vi "生成出厂配置.vi"(8 "error in":errorcluster) -> (0 "error out":errorcluster, 2 "ture?":bool)   [LabVIEW 2016]
panel:
  out "Numeric":i32
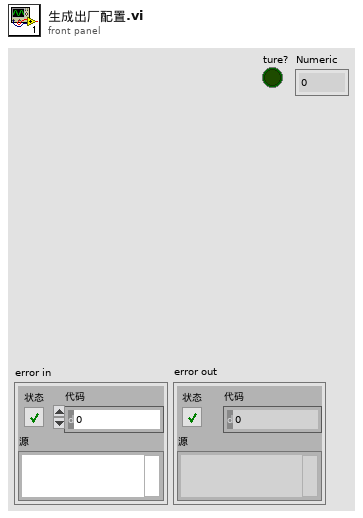
[diagram p1: front panel]
types:
  T1 = cluster{"byCmdType":u8, "bySubCmd":u8, "byPara":u8, "byAddr_h":u8, "byAddr_l":u8, "byAddr_ll":u8, "byLen_h":u8, "byLen_l":u8}
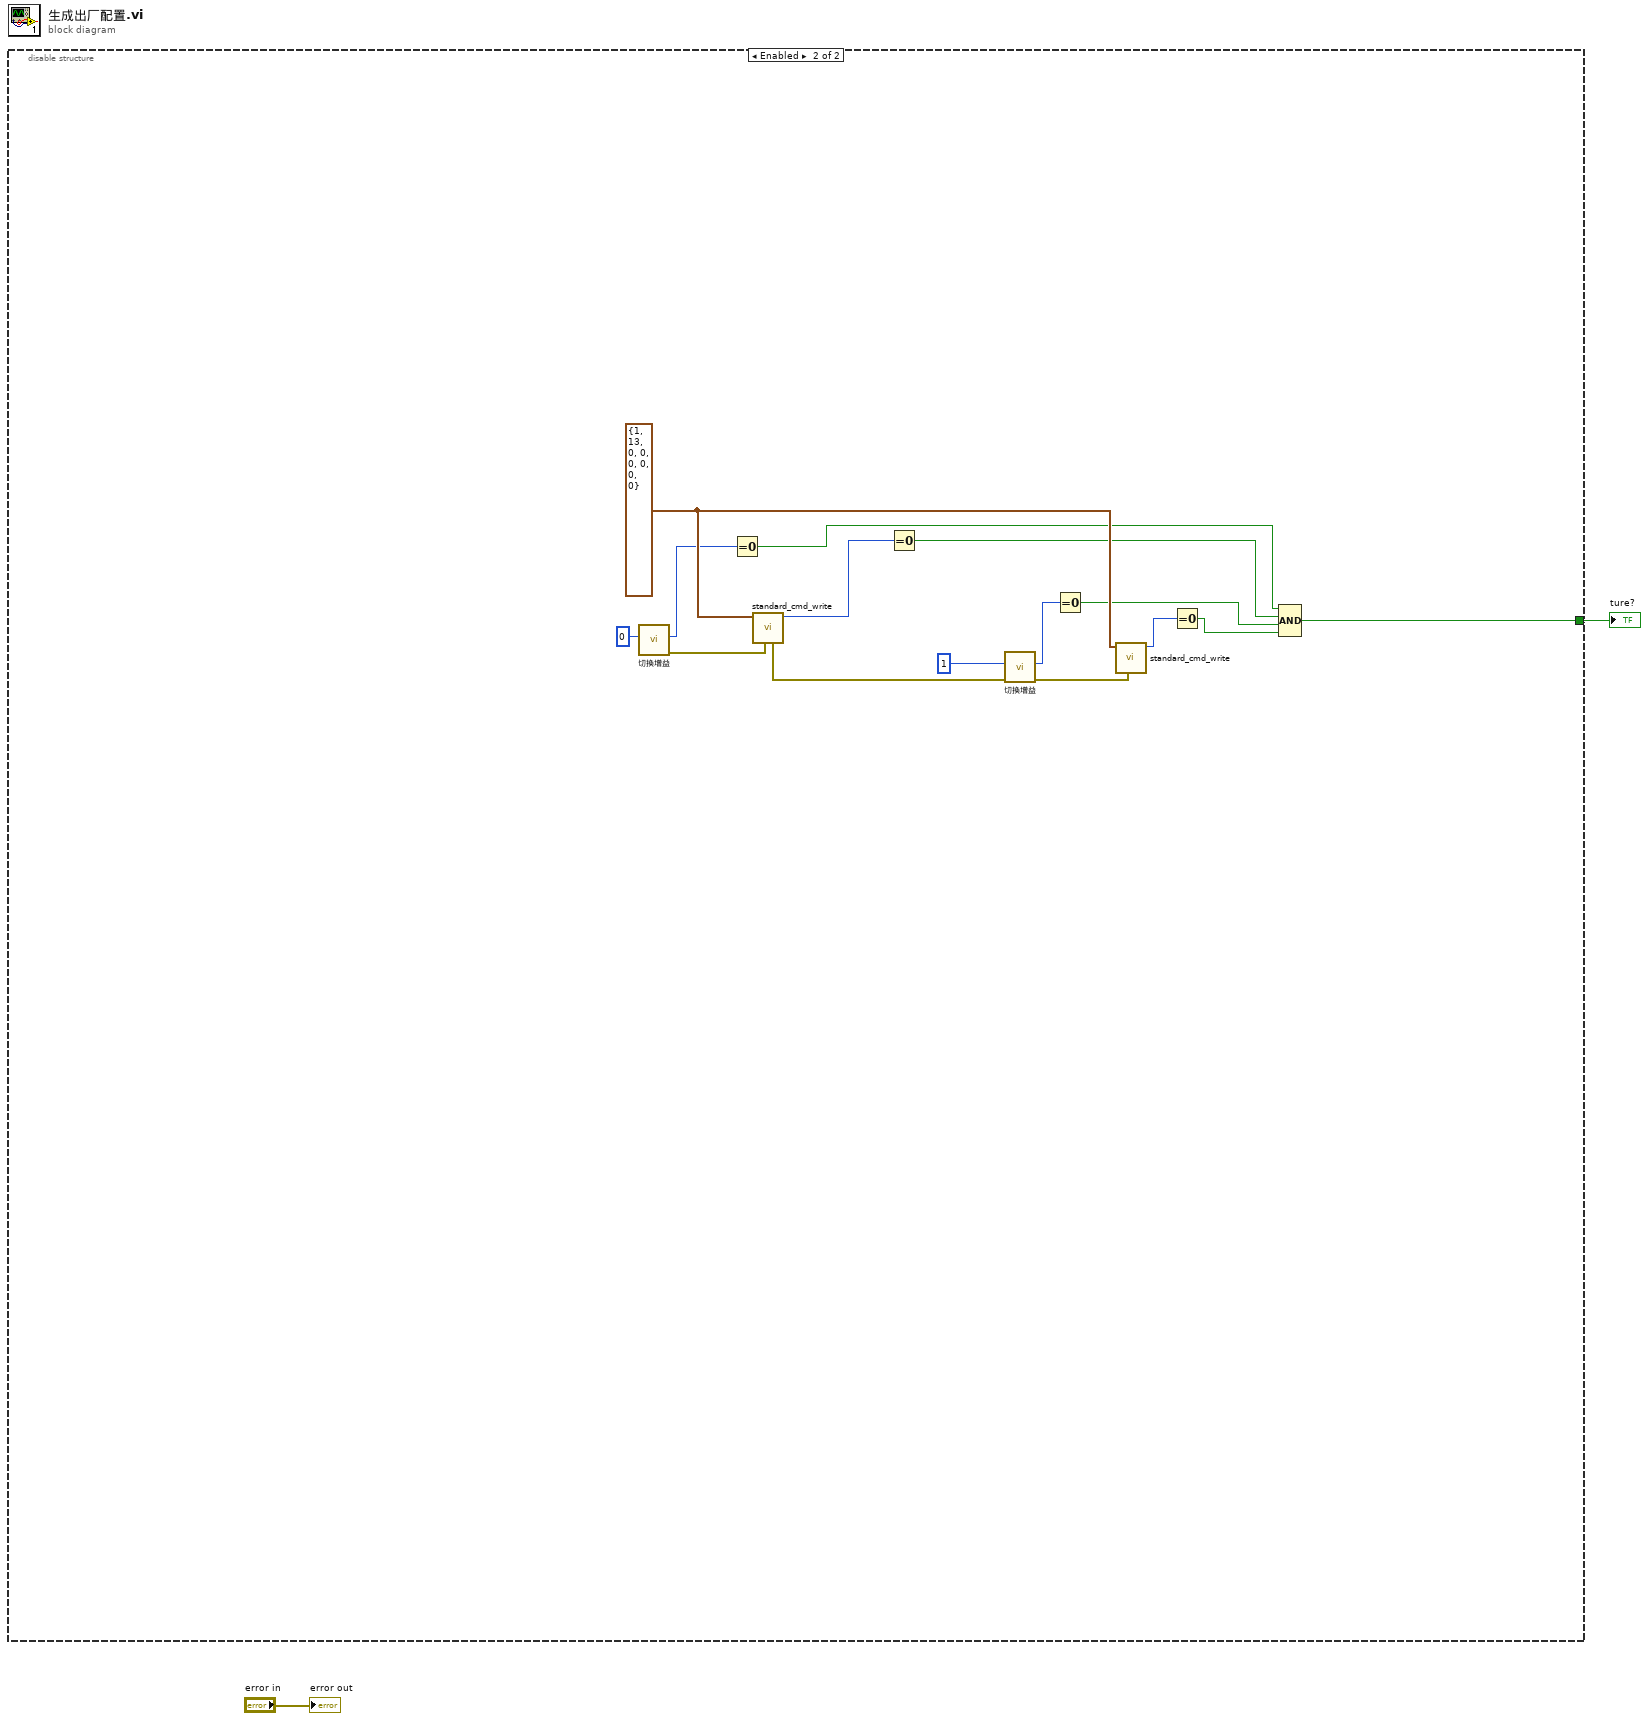
[diagram p0: block diagram]
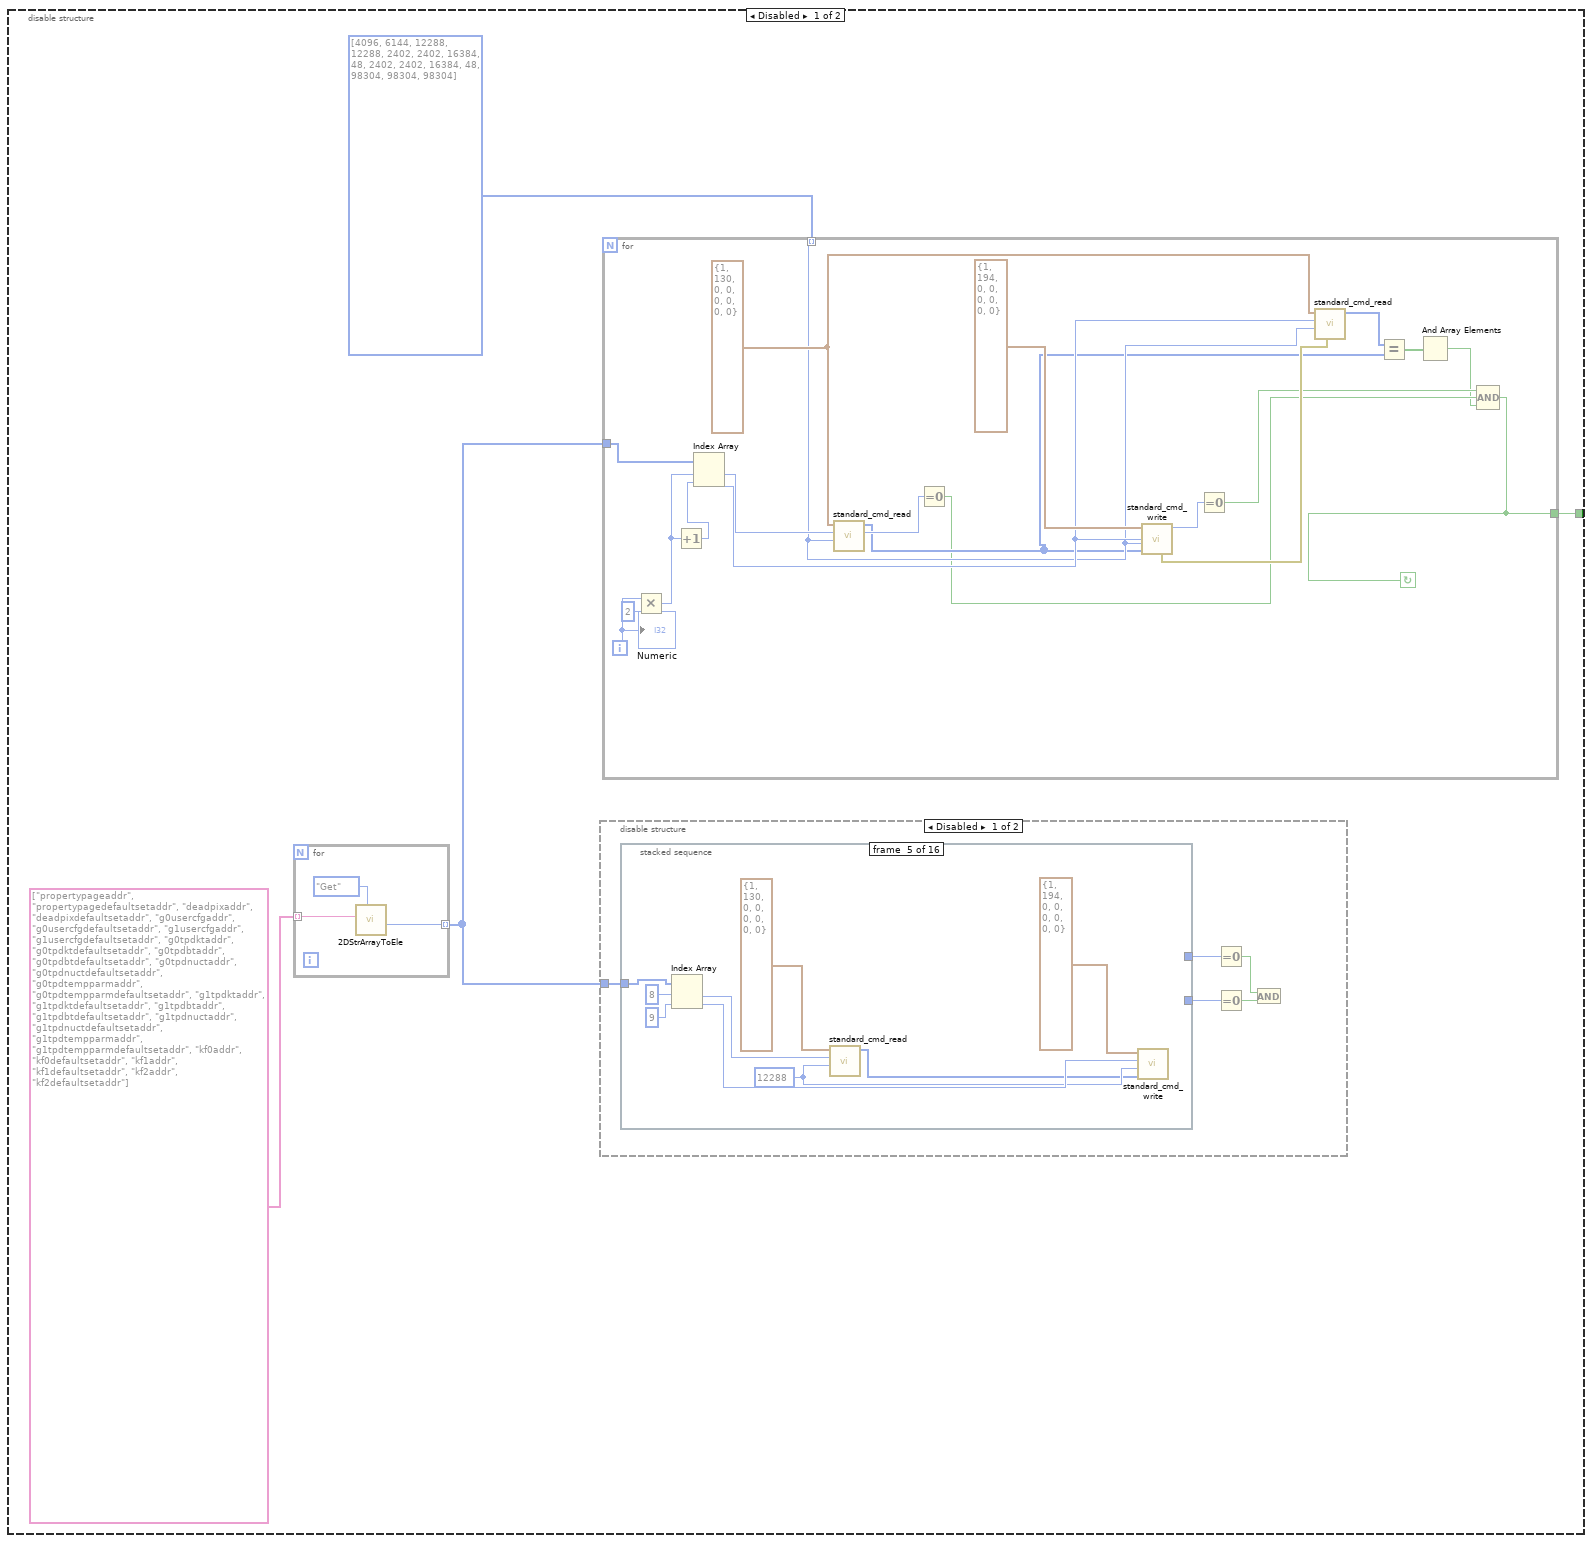
[diagram p2: hidden frame]
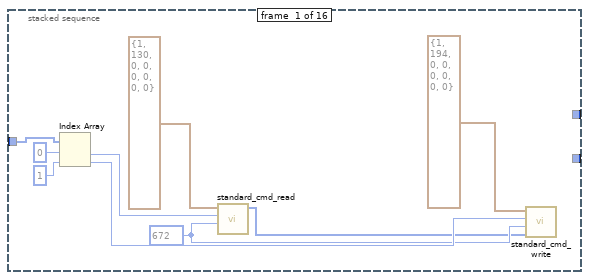
[diagram p3: hidden frame]
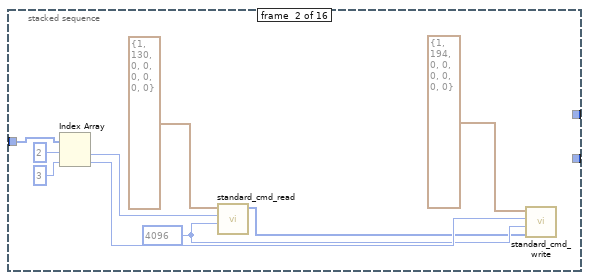
[diagram p4: hidden frame]
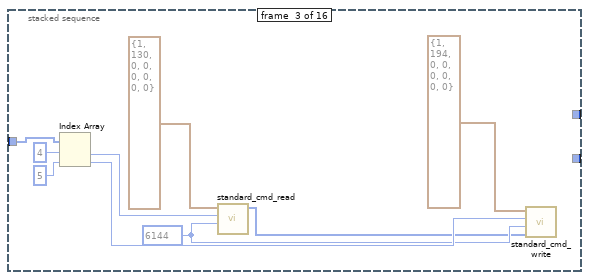
[diagram p5: hidden frame]
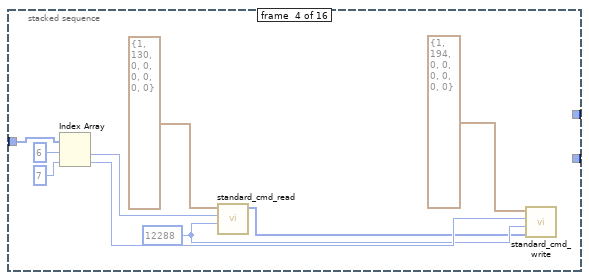
[diagram p6: hidden frame]
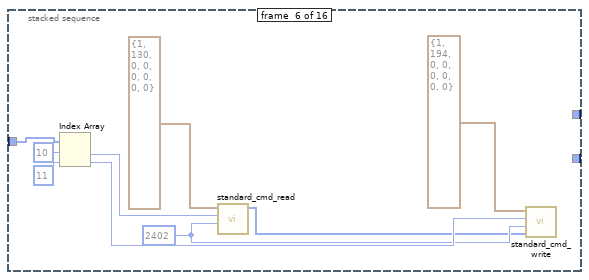
[diagram p7: hidden frame]
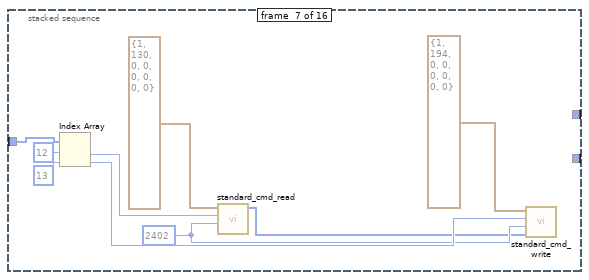
[diagram p8: hidden frame]
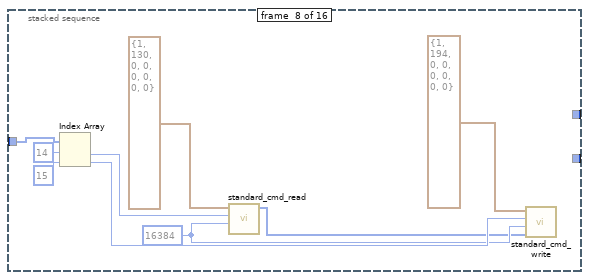
[diagram p9: hidden frame]
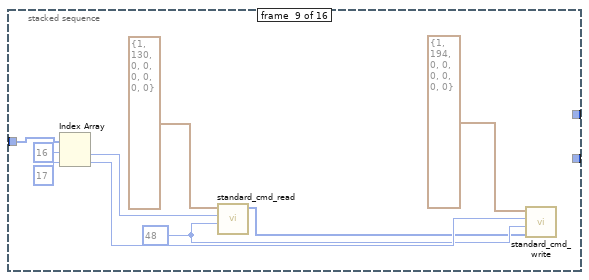
[diagram p10: hidden frame]
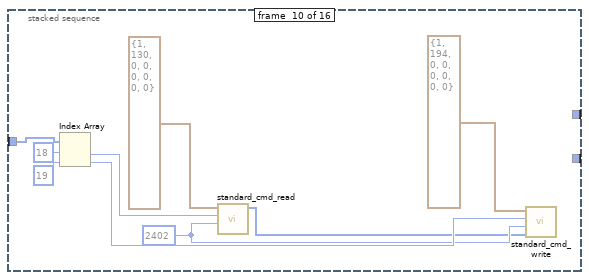
[diagram p11: hidden frame]
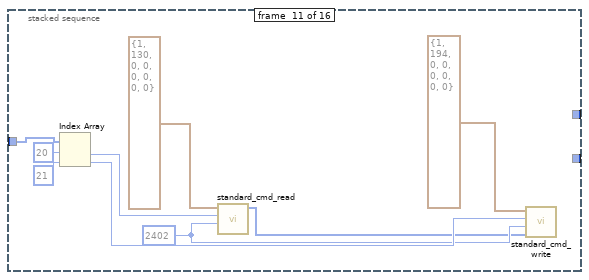
[diagram p12: hidden frame]
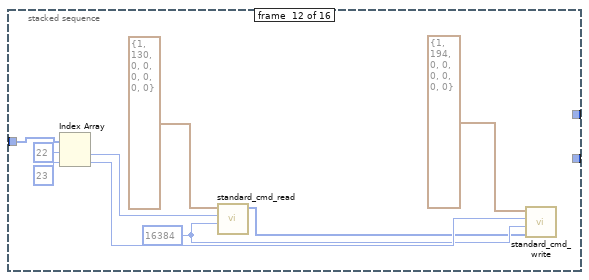
[diagram p13: hidden frame]
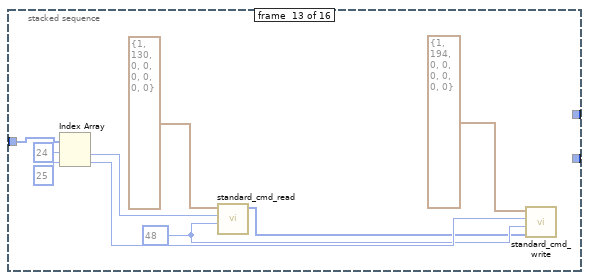
[diagram p14: hidden frame]
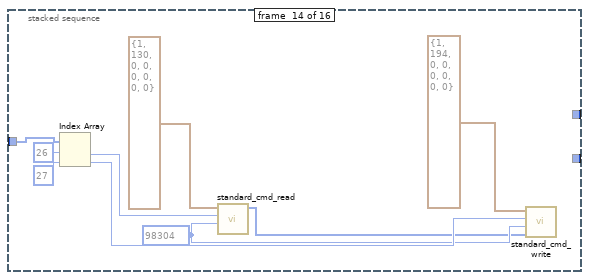
[diagram p15: hidden frame]
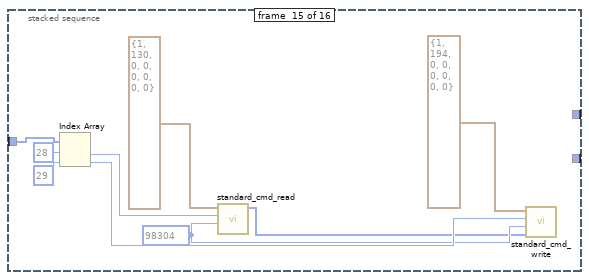
[diagram p16: hidden frame]
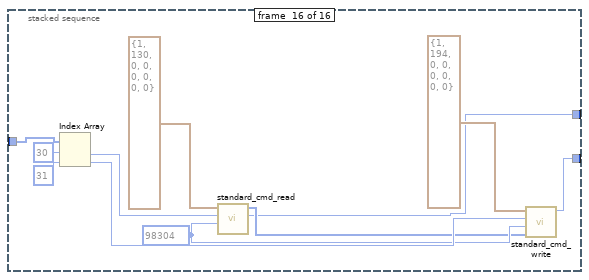
[diagram p17: hidden frame]
diagram:
  n1 = disable-structure shown="Enabled" {
    disable-tunnel: [w3 w181] -> w2
    frame Disabled {
      n2 = for {
        tunnel: string[] ["propertypageaddr", "propertypagedefaultsetaddr", "deadpixaddr", "deadpixdefaultsetaddr", "g0usercfgaddr", "g0usercfgdefaultsetaddr", "g1usercfgaddr", "g1usercfgdefaultsetaddr", "g0tpdktaddr", "g0tpdktdefaultsetaddr", "g0tpdbtaddr", "g0tpdbtdefaultsetaddr", "g0tpdnuctaddr", "g0tpdnuctdefaultsetaddr", "g0tpdtempparmaddr", "g0tpdtempparmdefaultsetaddr", "g1tpdktaddr", "g1tpdktdefaultsetaddr", "g1tpdbtaddr", "g1tpdbtdefaultsetaddr", "g1tpdnuctaddr", "g1tpdnuctdefaultsetaddr", "g1tpdtempparmaddr", "g1tpdtempparmdefaultsetaddr", "kf0addr", "kf0defaultsetaddr", "kf1addr", "kf1defaultsetaddr", "kf2addr", "kf2defaultsetaddr"] -> [w179] mode=indexing
        tunnel: [w178] -> w5 mode=indexing
        n3 = call "2DStrArrayToEle.vi"("Mothed"=enum16{"init", "Get", "Set", "Close"}."Get", "AddrName"=w179) -> ("Address"=w178:u32)  [unwired: 6 in, 3 out]
      }
      n4 = disable-structure shown="Disabled" {
        disable-tunnel: w5 -> [w7 _]
        frame Disabled {
          n5 = stacked-sequence {
            tunnel: w7 -> [w18 w27 w36 w45 w54 w63 w72 w81 w90 w99 w108 w117 w126 w135 w144 w155]
            tunnel: [_ _ _ _ _ _ _ _ _ _ _ _ _ _ _ w148] -> w11
            tunnel: [_ _ _ _ _ _ _ _ _ _ _ _ _ _ _ w147] -> w10
            frame #0 {
              w15 = 672
              n6 = Index Array(array=w18, index #1=0, index #2=1) -> (element #1=w17:u32, element #2=w16:u32)
              n7 = call "standard_cmd_read.vi"("dwLen"=w15, "dwAddr"=w17, "cmd_std_header_t"=T1 {"byCmdType"=1, "bySubCmd"=130, "byPara"=0, "byAddr_h"=0, "byAddr_l"=0, "byAddr_ll"=0, "byLen_h"=0, "byLen_l"=0}) -> ("data out"=w12:u8[])  [unwired: 6 in, 2 out]
              n8 = call "standard_cmd_write.vi"("data"=w12, "dwLen"=w15, "dwAddr"=w16, "cmd_std_header_t"=T1 {"byCmdType"=1, "bySubCmd"=194, "byPara"=0, "byAddr_h"=0, "byAddr_l"=0, "byAddr_ll"=0, "byLen_h"=0, "byLen_l"=0}) -> ()  [unwired: 6 in, 2 out]
            }
            frame #1 {
              w24 = 4096
              n9 = Index Array(array=w27, index #1=2, index #2=3) -> (element #1=w26:u32, element #2=w25:u32)
              n10 = call "standard_cmd_read.vi"("dwLen"=w24, "dwAddr"=w26, "cmd_std_header_t"=T1 {"byCmdType"=1, "bySubCmd"=130, "byPara"=0, "byAddr_h"=0, "byAddr_l"=0, "byAddr_ll"=0, "byLen_h"=0, "byLen_l"=0}) -> ("data out"=w21:u8[])  [unwired: 6 in, 2 out]
              n11 = call "standard_cmd_write.vi"("data"=w21, "dwLen"=w24, "dwAddr"=w25, "cmd_std_header_t"=T1 {"byCmdType"=1, "bySubCmd"=194, "byPara"=0, "byAddr_h"=0, "byAddr_l"=0, "byAddr_ll"=0, "byLen_h"=0, "byLen_l"=0}) -> ()  [unwired: 6 in, 2 out]
            }
            frame #2 {
              w33 = 6144
              n12 = Index Array(array=w36, index #1=4, index #2=5) -> (element #1=w35:u32, element #2=w34:u32)
              n13 = call "standard_cmd_read.vi"("dwLen"=w33, "dwAddr"=w35, "cmd_std_header_t"=T1 {"byCmdType"=1, "bySubCmd"=130, "byPara"=0, "byAddr_h"=0, "byAddr_l"=0, "byAddr_ll"=0, "byLen_h"=0, "byLen_l"=0}) -> ("data out"=w30:u8[])  [unwired: 6 in, 2 out]
              n14 = call "standard_cmd_write.vi"("data"=w30, "dwLen"=w33, "dwAddr"=w34, "cmd_std_header_t"=T1 {"byCmdType"=1, "bySubCmd"=194, "byPara"=0, "byAddr_h"=0, "byAddr_l"=0, "byAddr_ll"=0, "byLen_h"=0, "byLen_l"=0}) -> ()  [unwired: 6 in, 2 out]
            }
            frame #3 {
              w42 = 12288
              n15 = Index Array(array=w45, index #1=6, index #2=7) -> (element #1=w44:u32, element #2=w43:u32)
              n16 = call "standard_cmd_read.vi"("dwLen"=w42, "dwAddr"=w44, "cmd_std_header_t"=T1 {"byCmdType"=1, "bySubCmd"=130, "byPara"=0, "byAddr_h"=0, "byAddr_l"=0, "byAddr_ll"=0, "byLen_h"=0, "byLen_l"=0}) -> ("data out"=w39:u8[])  [unwired: 6 in, 2 out]
              n17 = call "standard_cmd_write.vi"("data"=w39, "dwLen"=w42, "dwAddr"=w43, "cmd_std_header_t"=T1 {"byCmdType"=1, "bySubCmd"=194, "byPara"=0, "byAddr_h"=0, "byAddr_l"=0, "byAddr_ll"=0, "byLen_h"=0, "byLen_l"=0}) -> ()  [unwired: 6 in, 2 out]
            }
            frame #4 {
              w51 = 12288
              n18 = Index Array(array=w54, index #1=8, index #2=9) -> (element #1=w53:u32, element #2=w52:u32)
              n19 = call "standard_cmd_read.vi"("dwLen"=w51, "dwAddr"=w53, "cmd_std_header_t"=T1 {"byCmdType"=1, "bySubCmd"=130, "byPara"=0, "byAddr_h"=0, "byAddr_l"=0, "byAddr_ll"=0, "byLen_h"=0, "byLen_l"=0}) -> ("data out"=w48:u8[])  [unwired: 6 in, 2 out]
              n20 = call "standard_cmd_write.vi"("data"=w48, "dwLen"=w51, "dwAddr"=w52, "cmd_std_header_t"=T1 {"byCmdType"=1, "bySubCmd"=194, "byPara"=0, "byAddr_h"=0, "byAddr_l"=0, "byAddr_ll"=0, "byLen_h"=0, "byLen_l"=0}) -> ()  [unwired: 6 in, 2 out]
            }
            frame #5 {
              w60 = 2402
              n21 = Index Array(array=w63, index #1=10, index #2=11) -> (element #1=w62:u32, element #2=w61:u32)
              n22 = call "standard_cmd_read.vi"("dwLen"=w60, "dwAddr"=w62, "cmd_std_header_t"=T1 {"byCmdType"=1, "bySubCmd"=130, "byPara"=0, "byAddr_h"=0, "byAddr_l"=0, "byAddr_ll"=0, "byLen_h"=0, "byLen_l"=0}) -> ("data out"=w57:u8[])  [unwired: 6 in, 2 out]
              n23 = call "standard_cmd_write.vi"("data"=w57, "dwLen"=w60, "dwAddr"=w61, "cmd_std_header_t"=T1 {"byCmdType"=1, "bySubCmd"=194, "byPara"=0, "byAddr_h"=0, "byAddr_l"=0, "byAddr_ll"=0, "byLen_h"=0, "byLen_l"=0}) -> ()  [unwired: 6 in, 2 out]
            }
            frame #6 {
              w69 = 2402
              n24 = Index Array(array=w72, index #1=12, index #2=13) -> (element #1=w71:u32, element #2=w70:u32)
              n25 = call "standard_cmd_read.vi"("dwLen"=w69, "dwAddr"=w71, "cmd_std_header_t"=T1 {"byCmdType"=1, "bySubCmd"=130, "byPara"=0, "byAddr_h"=0, "byAddr_l"=0, "byAddr_ll"=0, "byLen_h"=0, "byLen_l"=0}) -> ("data out"=w66:u8[])  [unwired: 6 in, 2 out]
              n26 = call "standard_cmd_write.vi"("data"=w66, "dwLen"=w69, "dwAddr"=w70, "cmd_std_header_t"=T1 {"byCmdType"=1, "bySubCmd"=194, "byPara"=0, "byAddr_h"=0, "byAddr_l"=0, "byAddr_ll"=0, "byLen_h"=0, "byLen_l"=0}) -> ()  [unwired: 6 in, 2 out]
            }
            frame #7 {
              w78 = 16384
              n27 = Index Array(array=w81, index #1=14, index #2=15) -> (element #1=w80:u32, element #2=w79:u32)
              n28 = call "standard_cmd_read.vi"("dwLen"=w78, "dwAddr"=w80, "cmd_std_header_t"=T1 {"byCmdType"=1, "bySubCmd"=130, "byPara"=0, "byAddr_h"=0, "byAddr_l"=0, "byAddr_ll"=0, "byLen_h"=0, "byLen_l"=0}) -> ("data out"=w75:u8[])  [unwired: 6 in, 2 out]
              n29 = call "standard_cmd_write.vi"("data"=w75, "dwLen"=w78, "dwAddr"=w79, "cmd_std_header_t"=T1 {"byCmdType"=1, "bySubCmd"=194, "byPara"=0, "byAddr_h"=0, "byAddr_l"=0, "byAddr_ll"=0, "byLen_h"=0, "byLen_l"=0}) -> ()  [unwired: 6 in, 2 out]
            }
            frame #8 {
              w87 = 48
              n30 = Index Array(array=w90, index #1=16, index #2=17) -> (element #1=w89:u32, element #2=w88:u32)
              n31 = call "standard_cmd_read.vi"("dwLen"=w87, "dwAddr"=w89, "cmd_std_header_t"=T1 {"byCmdType"=1, "bySubCmd"=130, "byPara"=0, "byAddr_h"=0, "byAddr_l"=0, "byAddr_ll"=0, "byLen_h"=0, "byLen_l"=0}) -> ("data out"=w84:u8[])  [unwired: 6 in, 2 out]
              n32 = call "standard_cmd_write.vi"("data"=w84, "dwLen"=w87, "dwAddr"=w88, "cmd_std_header_t"=T1 {"byCmdType"=1, "bySubCmd"=194, "byPara"=0, "byAddr_h"=0, "byAddr_l"=0, "byAddr_ll"=0, "byLen_h"=0, "byLen_l"=0}) -> ()  [unwired: 6 in, 2 out]
            }
            frame #9 {
              w96 = 2402
              n33 = Index Array(array=w99, index #1=18, index #2=19) -> (element #1=w98:u32, element #2=w97:u32)
              n34 = call "standard_cmd_read.vi"("dwLen"=w96, "dwAddr"=w98, "cmd_std_header_t"=T1 {"byCmdType"=1, "bySubCmd"=130, "byPara"=0, "byAddr_h"=0, "byAddr_l"=0, "byAddr_ll"=0, "byLen_h"=0, "byLen_l"=0}) -> ("data out"=w93:u8[])  [unwired: 6 in, 2 out]
              n35 = call "standard_cmd_write.vi"("data"=w93, "dwLen"=w96, "dwAddr"=w97, "cmd_std_header_t"=T1 {"byCmdType"=1, "bySubCmd"=194, "byPara"=0, "byAddr_h"=0, "byAddr_l"=0, "byAddr_ll"=0, "byLen_h"=0, "byLen_l"=0}) -> ()  [unwired: 6 in, 2 out]
            }
            frame #10 {
              w105 = 2402
              n36 = Index Array(array=w108, index #1=20, index #2=21) -> (element #1=w107:u32, element #2=w106:u32)
              n37 = call "standard_cmd_read.vi"("dwLen"=w105, "dwAddr"=w107, "cmd_std_header_t"=T1 {"byCmdType"=1, "bySubCmd"=130, "byPara"=0, "byAddr_h"=0, "byAddr_l"=0, "byAddr_ll"=0, "byLen_h"=0, "byLen_l"=0}) -> ("data out"=w102:u8[])  [unwired: 6 in, 2 out]
              n38 = call "standard_cmd_write.vi"("data"=w102, "dwLen"=w105, "dwAddr"=w106, "cmd_std_header_t"=T1 {"byCmdType"=1, "bySubCmd"=194, "byPara"=0, "byAddr_h"=0, "byAddr_l"=0, "byAddr_ll"=0, "byLen_h"=0, "byLen_l"=0}) -> ()  [unwired: 6 in, 2 out]
            }
            frame #11 {
              w114 = 16384
              n39 = Index Array(array=w117, index #1=22, index #2=23) -> (element #1=w116:u32, element #2=w115:u32)
              n40 = call "standard_cmd_read.vi"("dwLen"=w114, "dwAddr"=w116, "cmd_std_header_t"=T1 {"byCmdType"=1, "bySubCmd"=130, "byPara"=0, "byAddr_h"=0, "byAddr_l"=0, "byAddr_ll"=0, "byLen_h"=0, "byLen_l"=0}) -> ("data out"=w111:u8[])  [unwired: 6 in, 2 out]
              n41 = call "standard_cmd_write.vi"("data"=w111, "dwLen"=w114, "dwAddr"=w115, "cmd_std_header_t"=T1 {"byCmdType"=1, "bySubCmd"=194, "byPara"=0, "byAddr_h"=0, "byAddr_l"=0, "byAddr_ll"=0, "byLen_h"=0, "byLen_l"=0}) -> ()  [unwired: 6 in, 2 out]
            }
            frame #12 {
              w123 = 48
              n42 = Index Array(array=w126, index #1=24, index #2=25) -> (element #1=w125:u32, element #2=w124:u32)
              n43 = call "standard_cmd_read.vi"("dwLen"=w123, "dwAddr"=w125, "cmd_std_header_t"=T1 {"byCmdType"=1, "bySubCmd"=130, "byPara"=0, "byAddr_h"=0, "byAddr_l"=0, "byAddr_ll"=0, "byLen_h"=0, "byLen_l"=0}) -> ("data out"=w120:u8[])  [unwired: 6 in, 2 out]
              n44 = call "standard_cmd_write.vi"("data"=w120, "dwLen"=w123, "dwAddr"=w124, "cmd_std_header_t"=T1 {"byCmdType"=1, "bySubCmd"=194, "byPara"=0, "byAddr_h"=0, "byAddr_l"=0, "byAddr_ll"=0, "byLen_h"=0, "byLen_l"=0}) -> ()  [unwired: 6 in, 2 out]
            }
            frame #13 {
              w132 = 98304
              n45 = Index Array(array=w135, index #1=26, index #2=27) -> (element #1=w134:u32, element #2=w133:u32)
              n46 = call "standard_cmd_read.vi"("dwLen"=w132, "dwAddr"=w134, "cmd_std_header_t"=T1 {"byCmdType"=1, "bySubCmd"=130, "byPara"=0, "byAddr_h"=0, "byAddr_l"=0, "byAddr_ll"=0, "byLen_h"=0, "byLen_l"=0}) -> ("data out"=w129:u8[])  [unwired: 6 in, 2 out]
              n47 = call "standard_cmd_write.vi"("data"=w129, "dwLen"=w132, "dwAddr"=w133, "cmd_std_header_t"=T1 {"byCmdType"=1, "bySubCmd"=194, "byPara"=0, "byAddr_h"=0, "byAddr_l"=0, "byAddr_ll"=0, "byLen_h"=0, "byLen_l"=0}) -> ()  [unwired: 6 in, 2 out]
            }
            frame #14 {
              w141 = 98304
              n48 = Index Array(array=w144, index #1=28, index #2=29) -> (element #1=w143:u32, element #2=w142:u32)
              n49 = call "standard_cmd_read.vi"("dwLen"=w141, "dwAddr"=w143, "cmd_std_header_t"=T1 {"byCmdType"=1, "bySubCmd"=130, "byPara"=0, "byAddr_h"=0, "byAddr_l"=0, "byAddr_ll"=0, "byLen_h"=0, "byLen_l"=0}) -> ("data out"=w138:u8[])  [unwired: 6 in, 2 out]
              n50 = call "standard_cmd_write.vi"("data"=w138, "dwLen"=w141, "dwAddr"=w142, "cmd_std_header_t"=T1 {"byCmdType"=1, "bySubCmd"=194, "byPara"=0, "byAddr_h"=0, "byAddr_l"=0, "byAddr_ll"=0, "byLen_h"=0, "byLen_l"=0}) -> ()  [unwired: 6 in, 2 out]
            }
            frame #15 {
              w152 = 98304
              n51 = Index Array(array=w155, index #1=30, index #2=31) -> (element #1=w154:u32, element #2=w153:u32)
              n52 = call "standard_cmd_read.vi"("dwLen"=w152, "dwAddr"=w154, "cmd_std_header_t"=T1 {"byCmdType"=1, "bySubCmd"=130, "byPara"=0, "byAddr_h"=0, "byAddr_l"=0, "byAddr_ll"=0, "byLen_h"=0, "byLen_l"=0}) -> ("return"=w148:i32, "data out"=w149:u8[])  [unwired: 6 in, 1 out]
              n53 = call "standard_cmd_write.vi"("data"=w149, "dwLen"=w152, "dwAddr"=w153, "cmd_std_header_t"=T1 {"byCmdType"=1, "bySubCmd"=194, "byPara"=0, "byAddr_h"=0, "byAddr_l"=0, "byAddr_ll"=0, "byLen_h"=0, "byLen_l"=0}) -> ("return"=w147:i32)  [unwired: 6 in, 1 out]
            }
          }
          n54 = Equal To 0?(x=w11) -> (x = 0?=w8:bool)
          n55 = Equal To 0?(x=w10) -> (x = 0?=w9:bool)
          n56 = And(x=w8, y=w9) -> ()  [unwired: 1 out]
        }
        frame Enabled {
        }
      }
      n57 = for {
        tunnel: w5 -> [w177]
        tunnel: i32[] [4096, 6144, 12288, 12288, 2402, 2402, 16384, 48, 2402, 2402, 16384, 48, 98304, 98304, 98304] -> [w166] mode=indexing
        tunnel: [w158] -> w3
        i -> [w176]
        stop <- w158 continue-if-true
        w168 = T1 {"byCmdType"=1, "bySubCmd"=130, "byPara"=0, "byAddr_h"=0, "byAddr_l"=0, "byAddr_ll"=0, "byLen_h"=0, "byLen_l"=0} ("cmd_std_header_t")
        n58 = Multiply(x=w176, y=2) -> (x*y=w174:i32)
        n59 = Increment(x=w174) -> (x+1=w173:i32)
        n60 = Index Array(array=w177, index #1=w174, index #2=w173) -> (element #1=w170:u32, element #2=w167:u32)
        n61 = call "standard_cmd_read.vi"("dwLen"=w166, "dwAddr"=w170, "cmd_std_header_t"=w168) -> ("return"=w172:i32, "data out"=w163:u8[])  [unwired: 6 in, 1 out]
        n62 = Equal To 0?(x=w172) -> (x = 0?=w160:bool)
        n63 = call "standard_cmd_write.vi"("data"=w163, "dwLen"=w166, "dwAddr"=w167, "cmd_std_header_t"=T1 {"byCmdType"=1, "bySubCmd"=194, "byPara"=0, "byAddr_h"=0, "byAddr_l"=0, "byAddr_ll"=0, "byLen_h"=0, "byLen_l"=0}) -> ("return"=w171:i32, "error out"=w165:errorcluster)  [unwired: 6 in]
        n64 = Equal To 0?(x=w171) -> (x = 0?=w161:bool)
        n65 = call "standard_cmd_read.vi"("error in (no error)"=w165, "dwLen"=w166, "dwAddr"=w167, "cmd_std_header_t"=w168) -> ("data out"=w164:u8[])  [unwired: 5 in, 2 out]
        n66 = Equal?(x=w164, y=w163) -> (x = y?=w162:bool[])
        n67 = And Array Elements(Boolean array=w162) -> (logical AND=w159:bool)
        n68 = Compound Arithmetic op=AND(w161, w160, w159) -> (w158:bool)
        "Numeric" <- w176
      }
    }
    frame Enabled {
      w189 = T1 {"byCmdType"=1, "bySubCmd"=13, "byPara"=0, "byAddr_h"=0, "byAddr_l"=0, "byAddr_ll"=0, "byLen_h"=0, "byLen_l"=0} ("cmd_std_header_t")
      n69 = call "切换增益.vi"("增益"=u32 0) -> ("error out"=w194:errorcluster, "return"=w188:i32)  [unwired: 9 in]
      n70 = Equal To 0?(x=w188) -> (x = 0?=w185:bool)
      n71 = call "standard_cmd_write.vi"("error in (no error)"=w194, "cmd_std_header_t"=w189) -> ("return"=w195:i32, "error out"=w192:errorcluster)  [unwired: 8 in]
      n72 = Equal To 0?(x=w195) -> (x = 0?=w184:bool)
      n73 = call "切换增益.vi"("error in"=w192, "增益"=u32 1) -> ("error out"=w190:errorcluster, "return"=w187:i32)  [unwired: 8 in]
      n74 = Equal To 0?(x=w187) -> (x = 0?=w183:bool)
      n75 = call "standard_cmd_write.vi"("error in (no error)"=w190, "cmd_std_header_t"=w189) -> ("return"=w186:i32)  [unwired: 8 in, 1 out]
      n76 = Equal To 0?(x=w186) -> (x = 0?=w182:bool)
      n77 = Compound Arithmetic op=AND(w185, w184, w183, w182) -> (w181:bool)
    }
  }
  "ture?" <- w2
  "error out" <- "error in"
